vi "DependencyConstant.vi"   [LabVIEW 2020, in "OpenLvVision_OpenCv.lvlib"]
doc: "This VI makes sure the LabVIEW compile includes all necessary DLLs when you want to build an executable."
uses:
  OpenLvVision_OpenCv.lvlib
  Dlls/libopenblas.dll
  Dlls/OlvOpenCvWrapper.dll
  Dlls/opencv_world4110.dll
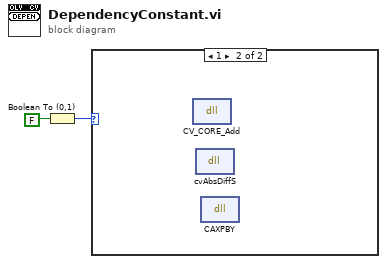
[diagram p0: block diagram]
diagram:
  n1 = Boolean To (0,1)(Boolean=FALSE) -> (0, 1=w2:i16)
  n2 = case shown="1" w2 {
    frame 0, Default {
    }
    frame 1 {
      n3 = dll-call lib="C:/Users/lukas/Downloads/OpenLvVision_OpenCv/SourceCode/LabView/OpenLvVision_OpenCv/Dlls/OlvOpenCvWrapper.dll" fn="CV_CORE_Add"() -> ()  [unwired: 4 in, 2 out]
      n4 = dll-call lib="C:/Users/lukas/Downloads/OpenLvVision_OpenCv/SourceCode/LabView/OpenLvVision_OpenCv/Dlls/opencv_world4110.dll" fn="cvAbsDiffS"() -> ()  [unwired: 4 in, 2 out]
      n5 = dll-call lib="C:/Users/lukas/Downloads/OpenLvVision_OpenCv/SourceCode/LabView/OpenLvVision_OpenCv/Dlls/libopenblas.dll" fn="CAXPBY"() -> ()  [unwired: 4 in, 2 out]
    }
  }
